vi "Error.vi"(10 "error in (no error)":errorcluster, 11 "PQ Result  In":refnum<class "PQ Result.lvclass">) -> (2 "error out":errorcluster, 3 "PQ Result":refnum<class "PQ Result.lvclass">)   [LabVIEW 2015, in "PQ Result.lvclass"]
uses:
  PQ Result.lvclass
  PQ Result.lvclass/PQ Result.ctl
  Connection/libpq.dll
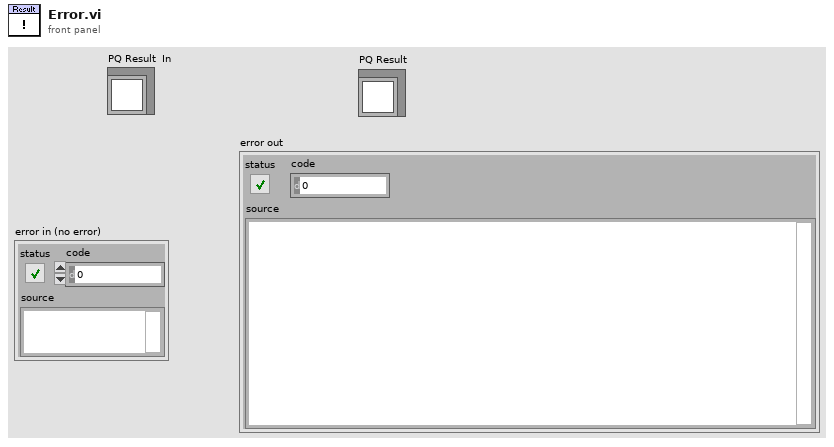
[diagram p1: front panel]
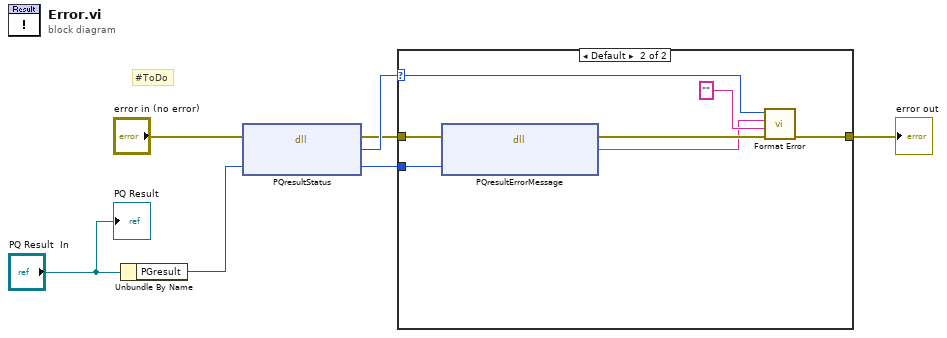
[diagram p0: block diagram]
diagram:
  # "#ToDo"
  n1 = Unbundle By Name("PQ Result  In") -> ("PGresult"=w6:u32)
  n2 = dll-call lib="C:/PQ/Connection/libpq.dll" fn="PQresultStatus" ("libpq.*:PQstatus")(error in="error in (no error)", "PGresult"=w6) -> (error out=w3:errorcluster, "PQstatus"=w5:u32, "PGresult"=w1:u32)  [unwired: 2 in, 1 out]
  n3 = case shown="Default" w5 {
    selector: w5 -> [_ w10]
    tunnel: w3 -> [w8 w15]
    tunnel: w1 -> [_ w14]
    tunnel: [w8 w12] -> w7
    frame 0 {
    }
    frame Default {
      n4 = dll-call lib="C:/PQ/Connection/libpq.dll" fn="PQresultErrorMessage" ("libpq.*:PQerrorMessage")(error in=w15, "PGresult"=w14) -> (error out=w11:errorcluster, "PQerrorMessage"=w9:string)  [unwired: 3 in, 1 out]
      n5 = call "Format Error.vi"("error in (no error)"=w11, "Additional source description"="", "error message"=w9, "error code"=w10) -> ("error out"=w12:errorcluster)  [unwired: 7 in]
    }
  }
  "error out" <- w7
  "PQ Result" <- "PQ Result  In"
